vi "Referenzabweichung berechnen.vi"(7 "Referenz in":sgl, 10 "Boolesch":bool, 11 "Array (Eingang)":string[][](array[string])) -> (3 "Array (Ausgang)":string[][](array[string]))   [LabVIEW 2020, in "EPA 1065.lvlib" / "HovaCAL Interference verificaton.lvlib"]
uses:
  HovaCAL Interference verificaton.lvlib
  Linearisierung V2/AutoLin Protokoll/AutoLin Protokoll.lvlib
  Linearisierung V2/SpanEinstellungen/SpanEinstellungen.lvlib
  Allgemein/allgemeine Sub-VIs.lvlib
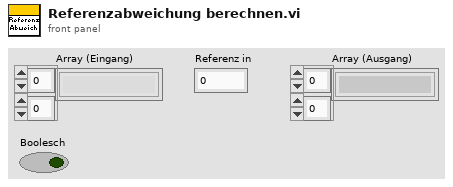
[diagram p1: front panel]
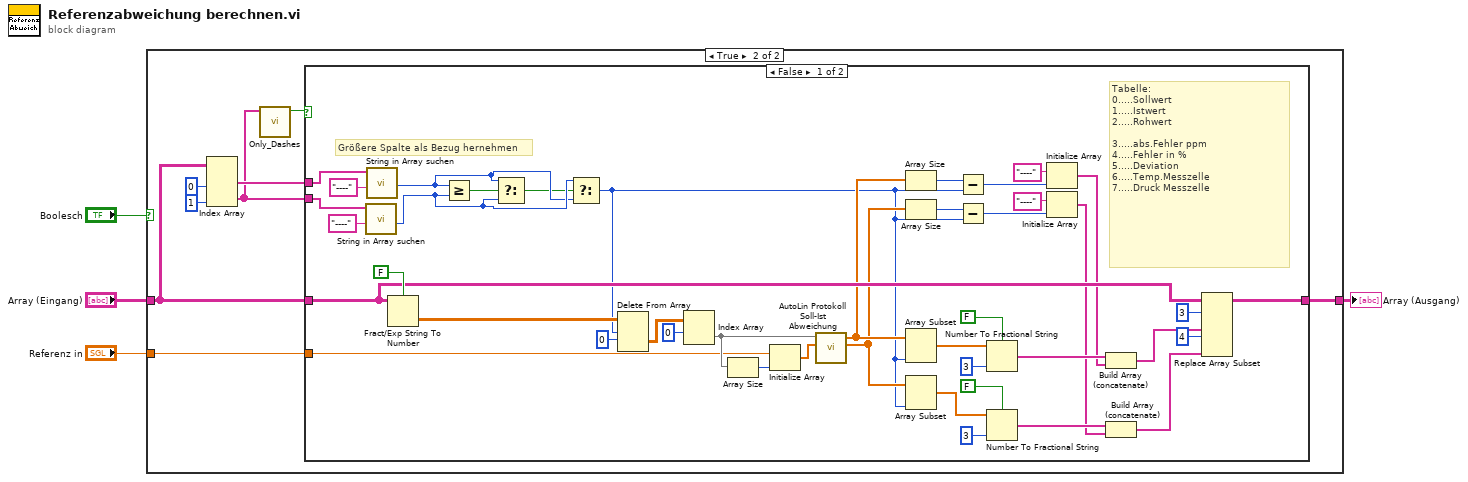
[diagram p0: block diagram]
diagram:
  n1 = case shown="True" "Boolesch" {
    tunnel: "Array (Eingang)" -> [w5 w9]
    tunnel: [w5 w12] -> w4
    tunnel: "Referenz in" -> [_ w13]
    frame False {
    }
    frame True {
      n2 = Index Array(array=w9, index (col) #1=0 ("Deaktivierter Index (Spalte)"), index (col) #2=1 ("Index (Spalte)")) -> (element #1=w7:string[], element #2=w6:string[])  [unwired: 2 in]
      n3 = call "Only_Dashes.vi"("Eingabetabelle"=w6) -> ("Dashes_only"=w8:bool)  [unwired: 10 in]
      n4 = case shown="False" w8 {
        tunnel: w13 -> [w50 _]
        tunnel: [w44 w55] -> w12
        tunnel: w9 -> [w43 w55]
        tunnel: w7 -> [w36 _]
        tunnel: w6 -> [w35 _]
        frame False {
          # "Größere Spalte als Bezug hernehmen"
          # "Tabelle:\n0.....Sollwert\n1.....Istwert\n2.....Rohwert\n\n3.....abs.Fehler ppm\n4.....Fehler in %\n5.....Deviation\n6.....Temp.Messzelle\n7.....Druck Messzelle"
          n5 = call "String in Array suchen.vi"("Nach String/Zeichen suchen (-)"="----", "String-Array"=w35) -> ("Index"=w39:i32)  [unwired: 7 in, 2 out]
          n6 = call "String in Array suchen.vi"("Nach String/Zeichen suchen (-)"="----", "String-Array"=w36) -> ("Index"=w38:i32)  [unwired: 7 in, 2 out]
          n7 = Fract/Exp String To Number(use system decimal point (T)=FALSE ("Systemdezimalzeichen verwenden (T)"), string=w43) -> (number=w34:dbl[][])  [unwired: 2 in, 1 out]
          n8 = Greater Or Equal?(x=w38, y=w39) -> (x >= y?=w37:bool)
          n9 = Select(t=w38, s=w37, f=w39) -> (s? t:f=w24:i32)
          n10 = Select(t=w39, s=w37, f=w38) -> ()  [unwired: 1 out]
          n11 = Delete From Array(array=w34, length=w24, index (row)=0 ("Index (Zeile)")) -> (deleted portion=w33:dbl[][])  [unwired: 1 in, 1 out]
          n12 = Index Array(array=w33, index (row)=0 ("Index (Zeile)")) -> (element=w52:dbl[])  [unwired: 1 in]
          n13 = Array Size(array=w52) -> (size(s)=w51:i32)
          n14 = Initialize Array(w50, w51) -> (w49:sgl[])
          n15 = call "AutoLin Protokoll Soll-Ist Abweichung.vi"("Istwerte (ppm)"=w49, "Sollwerte (ppm)"=w52) -> ("% vom Sollwert"=w25:sgl[], "abs. Fehler (ppm)"=w26:sgl[])  [unwired: 7 in, 1 out]
          n16 = Array Size(array=w26) -> (size(s)=w32:i32)
          n17 = Array Size(array=w25) -> (size(s)=w31:i32)
          n18 = Array Subset(array=w26, length=w24) -> (w23:sgl[])  [unwired: 1 in]
          n19 = Array Subset(array=w25, length=w24) -> (w22:sgl[])  [unwired: 1 in]
          n20 = Subtract(x=w32, y=w24) -> (x-y=w29:i32)
          n21 = Subtract(x=w31, y=w24) -> (x-y=w27:i32)
          n22 = Number To Fractional String(use system decimal point (T)=FALSE ("Systemdezimalzeichen verwenden (T)"), number=w23, precision (6)=i16 3 ("Genauigkeit (6)")) -> (F-format string=w21:string[])  [unwired: 1 in]
          n23 = Number To Fractional String(use system decimal point (T)=FALSE ("Systemdezimalzeichen verwenden (T)"), number=w22, precision (6)=i16 3 ("Genauigkeit (6)")) -> (F-format string=w19:string[])  [unwired: 1 in]
          n24 = Initialize Array("----" ("Nach String/Zeichen suchen (-)"), w29) -> (w20:string[])
          n25 = Initialize Array("----" ("Nach String/Zeichen suchen (-)"), w27) -> (w18:string[])
          n26 = Build Array (concatenate)(w21, w20) -> (w17:string[])
          n27 = Build Array (concatenate)(w19, w18) -> (w16:string[])
          n28 = Replace Array Subset(array=w43, new element #1=w17, index (row) #1=3 ("Deaktivierter Index (Spalte)"), new element #2=w16, index (row) #2=4 ("Index (Spalte)")) -> (w44:string[][])  [unwired: 2 in]
        }
        frame True {
        }
      }
    }
  }
  "Array (Ausgang)" <- w4
